vi "Shutdown Core.vi"(8 "error in (no error)":errorcluster, 11 "Abstract Log Consumer in":refnum<class "Abstract Log Consumer.lvclass">) -> (0 "error out":errorcluster, 3 "Abstract Log Consumer out":refnum<class "Abstract Log Consumer.lvclass">)   [LabVIEW 2020]
uses:
  Abstract Log Consumer.lvclass
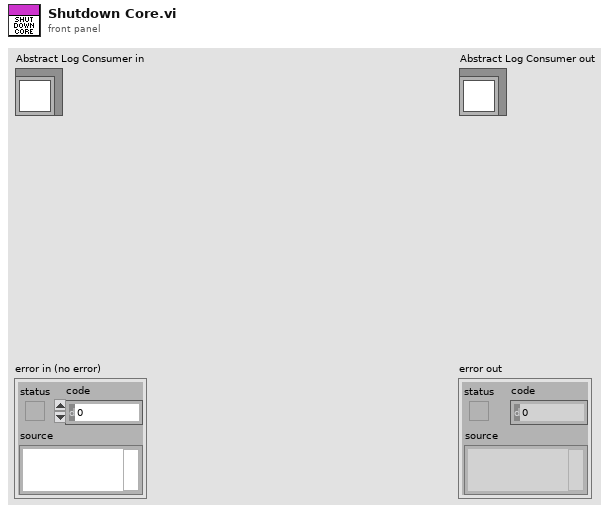
[diagram p1: front panel]
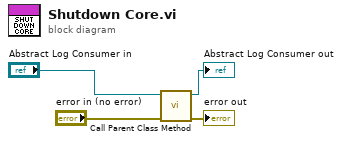
[diagram p0: block diagram]
diagram:
  n1 = call-parent "Call Parent Class Method"("error in (no error)"="error in (no error)", "Abstract Consumer in"="Abstract Log Consumer in") -> ("error out"=→"error out":errorcluster, "Abstract Consumer out"=→"Abstract Log Consumer out":refnum<class "Abstract Log Consumer.lvclass">)  [unwired: 8 in]
